vi "Actor Core.vi"(8 "error in":errorcluster, 11 "Normal Active Station View In":refnum<class "Normal Active Option View.lvclass">) -> (0 "error out":errorcluster, 3 "Actor out":refnum<class "Actor.lvclass">)   [LabVIEW 2019, in "Normal Active Option View.lvclass"]
doc: "(<B>Filename</B>: Actor Framework.lvlib:Actor.lvclass:Actor Core.vi)\n\nReceives messages to the actor, reacts to them, and initiates any error handling that may shut the actor down.\n\nDescendant classes may override this VI to append parallel tasks for the actor to complete while it handles messages. Overrides use the Call Parent Method node.\n\n<License>\nCopyright © 2017 Composed Systems, LLC | All rights reserved\nwww.composed.io\n\nAuthor: Ethan Stern <ethan.stern@composed.io>\n\nThis software is provided \"AS IS\" WITHOUT WARRANTIES, either express or implied, AND IS FOR EDUCATIONAL PURPOSES ONLY.\n</License>"
uses:
  <vilib>/gpm_packages/@cs/Car-wash/Source/Normal Active Station View/Normal Active Station View/Normal Active Option View.lvclass
  <vilib>/gpm_packages/@cs/Car-wash/Source/Active Station View Definition/Active Station View Definition/Active Option View Definition.lvclass
  <vilib>/gpm_packages/@cs/mva-core/Source/IObserver/IObserver/IObserver.lvclass
  C:/Program Files/National Instruments/LabVIEW 2019/vi.lib/gpm_packages/@cs/composed-car-wash/Source/Active Station View Definition/Active Station View Definition/Active Option View Definition.lvclass
  C:/Program Files/National Instruments/LabVIEW 2019/vi.lib/gpm_packages/@cs/mva-viewable/Source/IViewable/IViewable/IViewable.lvclass
  C:/Program Files/National Instruments/LabVIEW 2019/vi.lib/gpm_packages/@cs/mva-viewable/Source/ActorEvents/IEventAggregator/IEventAggregator.lvclass
  C:/Program Files/National Instruments/LabVIEW 2019/vi.lib/gpm_packages/@cs/mva-core/Source/IObserver/IObserver/IObserver.lvclass
  C:/Program Files/National Instruments/LabVIEW 2019/vi.lib/ActorFramework/Actor/Actor.lvclass
  <vilib>/ActorFramework/Actor/Actor.lvclass
panel:
  out "Vehicle Out of Position":bool
  out "Air Dry":bool
  out "Tire Shine Foam":bool
  out "Spot Free Rinse":bool
  out "Low Pressure Wax":bool
  out "High Pressure Wash":bool
  out "Pre-Soak":bool
  out "Bug Remover":bool
  out "Under Body Wash":bool
  # "Car Wash Indicators"
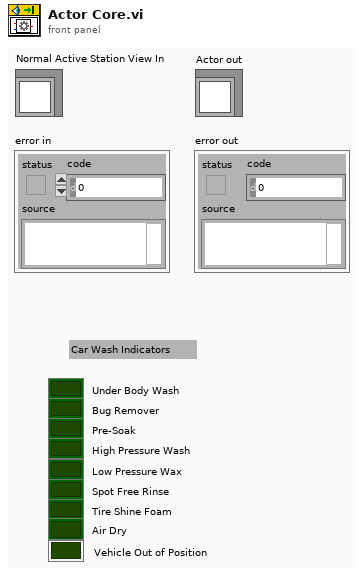
[diagram p1: front panel]
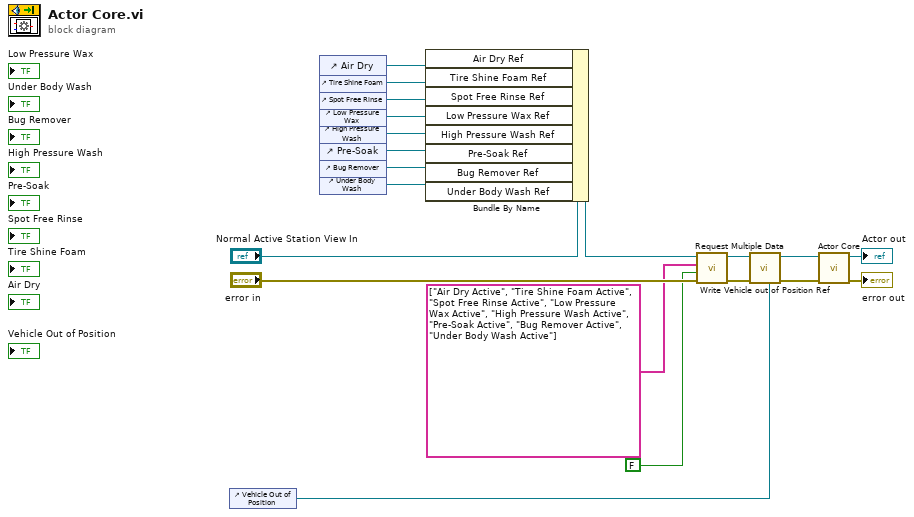
[diagram p0: block diagram]
diagram:
  n1 = control-ref of="Vehicle Out of Position"() -> (w16:refnum<vi>)
  n2 = control-ref of="Air Dry"() -> (w10:refnum<vi>)
  n3 = control-ref of="Tire Shine Foam"() -> (w9:refnum<vi>)
  n4 = control-ref of="Spot Free Rinse"() -> (w8:refnum<vi>)
  n5 = control-ref of="Low Pressure Wax"() -> (w7:refnum<vi>)
  n6 = control-ref of="High Pressure Wash"() -> (w6:refnum<vi>)
  n7 = control-ref of="Pre-Soak"() -> (w5:refnum<vi>)
  n8 = control-ref of="Bug Remover"() -> (w4:refnum<vi>)
  n9 = control-ref of="Under Body Wash"() -> (w3:refnum<vi>)
  n10 = Bundle By Name(cluster="Normal Active Station View In", "Air Dry Ref"=w10, "Tire Shine Foam Ref"=w9, "Spot Free Rinse Ref"=w8, "Low Pressure Wax Ref"=w7, "High Pressure Wash Ref"=w6, "Pre-Soak Ref"=w5, "Bug Remover Ref"=w4, "Under Body Wash Ref"=w3) -> (w11:refnum<class "Normal Active Option View.lvclass">)
  n11 = call <vilib>:"Request Multiple Data.vi"("error in (no error)"="error in", "Data Type"=FALSE, "Datum Names"=string[] ["Air Dry Active", "Tire Shine Foam Active", "Spot Free Rinse Active", "Low Pressure Wax Active", "High Pressure Wash Active", "Pre-Soak Active", "Bug Remover Active", "Under Body Wash Active"], "IObserver in"=w11) -> ("error out"=w13:errorcluster, "IObserver out"=w15:refnum<class "Normal Active Option View.lvclass">)  [unwired: 5 in, 1 out]
  n12 = call <vilib>:"Write Vehicle out of Position Ref.vi"("Vehicle Out of Position Ref"=w16, "Active Station View Definition in"=w15) -> ("Active Station View Definition out"=w17:refnum<class "Normal Active Option View.lvclass">)  [unwired: 9 in]
  n13 = call-parent "Actor Core.vi"("error in"=w13, "Active Station View Definition In"=w17) -> ("error out"=→"error out":errorcluster, "Actor out"=→"Actor out":refnum<class "Actor.lvclass">)  [unwired: 8 in]
